vi "LMT.API_TEMPLATE.vi"(8 "error in (no error)":errorcluster, 10 "Data":T1, 11 "LMT":refnum<class "LMT.lvclass">) -> (0 "error out":errorcluster, 3 "LMT out":refnum<class "LMT.lvclass">)   [LabVIEW 2017, in "LMT.lvclass"]
doc: "---------------------------------------------------------------\nJKI State Machine Objects™\nhttp://jki.net/state-machine-objects/\nCopyright (C) 2005-2015, JKI <info@jki.net>\nALL RIGHTS RESERVEDJKI State Machine Objects (SMO) 1.0.0.5\nJKI - JKI\nCopyright (c) 2016, JKI"
uses:
  LMT.lvclass
  Typedefs/Data.ctl
  Typedefs/API Inputs--Cluster.ctl
panel:
  # "For instructions on how to use the JKI State Machine Objects, examples and video tutorials, visit:\nhttp://jki.net/state-machine-objects/\n\nJKI State Machine Objects™\nhttp://jki.net/state-machine-objects/\nCopyright (C) 2005-2015, JKI <info@jki.net>\nALL RIGHTS RESERVED"
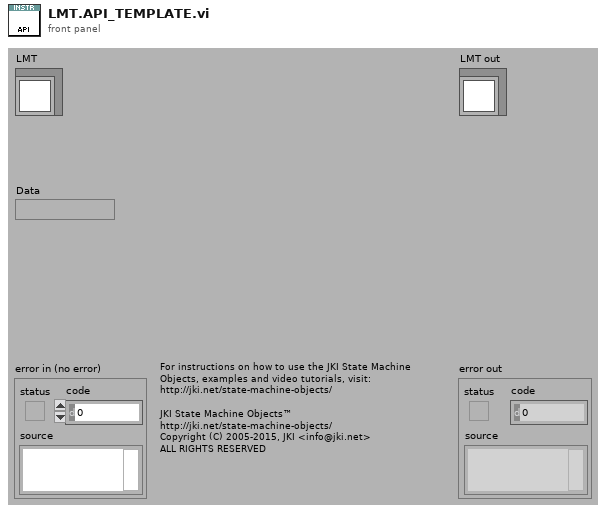
[diagram p1: front panel]
types:
  T1 = typedef "LMT.lvclass/Data.ctl" = string
  T2 = typedef "LMT.lvclass/API Inputs--Cluster.ctl" = cluster{"Data":T1}
  T3 = typedef "LMT.lvclass/PrivateEvents--Cluster.ctl" = cluster{"AsyncMethod":refnum<user-event>}
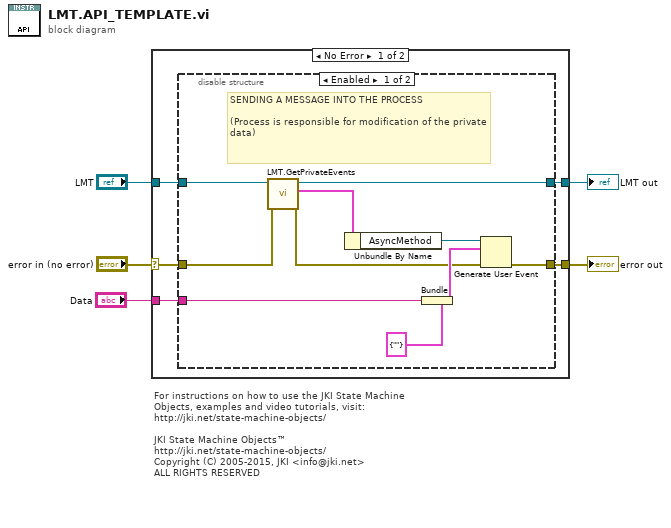
[diagram p0: block diagram]
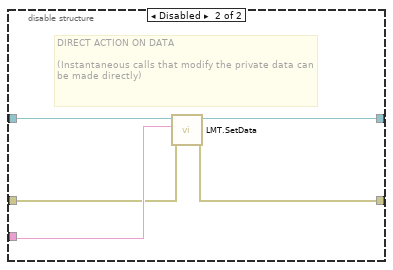
[diagram p2: hidden frame]
diagram:
  # "For instructions on how to use the JKI State Machine Objects, examples and video tutorials, visit:\nhttp://jki.net/state-machine-objects/\n\nJKI State Machine Objects™\nhttp://jki.net/state-machine-objects/\nCopyright (C) 2005-2015, JKI <info@jki.net>\nALL RIGHTS RESERVED"
  n1 = case shown="No Error" "error in (no error)" {
    selector: "error in (no error)" -> [w7 w26]
    tunnel: "LMT" -> [w8 w27]
    tunnel: [w9 w26] -> w4
    tunnel: [w6 w27] -> w3
    tunnel: "Data" -> [w10 _]
    frame No Error {
      n2 = disable-structure shown="Enabled" {
        disable-tunnel: w10 -> [w20 w24]
        disable-tunnel: [w19 w22] -> w9
        disable-tunnel: w8 -> [w15 w25]
        disable-tunnel: w7 -> [w14 w23]
        disable-tunnel: [w12 w21] -> w6
        frame Enabled {
          # "SENDING A MESSAGE INTO THE PROCESS\n\n(Process is responsible for modification of the private data)"
          n3 = call "LMT.GetPrivateEvents.vi"("error in (no error)"=w14, "LMT"=w15) -> ("error out"=w13:errorcluster, "Private Events"=w11:T3, "LMT out"=w12:refnum<class "LMT.lvclass">)  [unwired: 7 in]
          n4 = Unbundle By Name(w11) -> ("AsyncMethod"=w18:refnum<user-event>)
          n5 = Bundle(cluster=T2 {"Data"=""} ("event data"), "Data"=w20) -> (w16:T2)
          n6 = Generate User Event(user event=w18, event data cluster=w16, error in=w13) -> (error out=w19:errorcluster)  [unwired: 1 in, 1 out]
        }
        frame Disabled {
          # "DIRECT ACTION ON DATA\n\n(Instantaneous calls that modify the private data can be made directly)"
          n7 = call-dynamic "LMT.SetData.vi"("error in (no error)"=w23, "Data"=w24, "LMT"=w25) -> ("error out"=w22:errorcluster, "LMT out"=w21:refnum<class "LMT.lvclass">)  [unwired: 7 in]
        }
      }
    }
    frame Error {
    }
  }
  "error out" <- w4
  "LMT out" <- w3
